vi "GetPhysicalChannelArray.vi"(8 "error in (no error)":errorcluster, 11 "JSON Text":string) -> (0 "error out":errorcluster, 3 "PhysicalChannels Array":string[](array[string]) caption="<JSON>Elements")   [LabVIEW 2017]
uses:
  <vilib>/JDP Science/JSONtext/JSONtext.lvlib
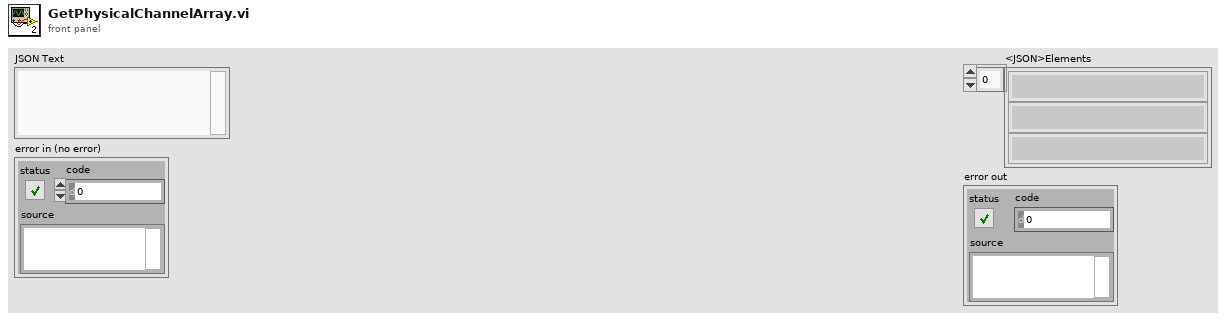
[diagram p1: front panel]
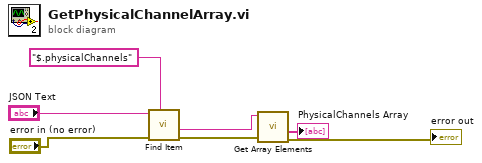
[diagram p0: block diagram]
diagram:
  n1 = call <vilib>:"Find Item.vi"("$Path or Item Name"="$.physicalChannels", "error in (no error)"="error in (no error)", "JSON"="JSON Text") -> ("error out"=w3:errorcluster, "<JSON>"=w4:string)  [unwired: 5 in, 2 out]
  n2 = call <vilib>:"Get Array Elements.vi"("error in (no error)"=w3, "JSON"=w4) -> ("error out"=→"error out":errorcluster, "<JSON>"=→"PhysicalChannels Array":string[])  [unwired: 7 in, 1 out]
